vi "SetState.vi"(8 "Error In":errorcluster, 10 "State":bool, 11 "reference in":refnum<class "VdDigitalControl_DAQmx.lvclass">) -> (0 "Error Out":errorcluster, 3 "reference in":refnum<class "VdDigitalControl_DAQmx.lvclass">)   [LabVIEW 2020, in "VdDigitalControl_DAQmx.lvclass"]
uses:
  VdDigitalControl_DAQmx.lvclass
  <vilib>/DAQmx/write.llb/DAQmx Write (Digital Bool 1Line 1Point).vi
  <vilib>/DAQmx/miscellaneous.llb/DAQmx Fill In Error Info.vi
  VdDigitalControl_class/VdDigitalControl.lvclass
  VdDigitalControl_DAQmx.lvclass/VdDigitalControl_DAQmx.ctl
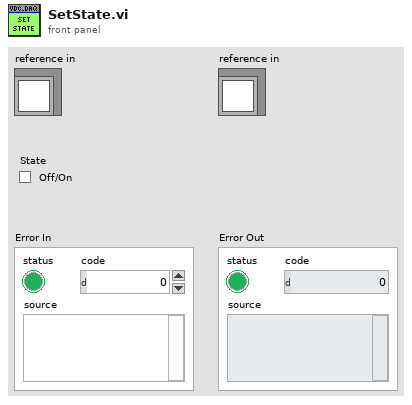
[diagram p1: front panel]
types:
  T1 = typedef "VdDigitalControl_DAQmx.lvclass/ObjectAttributes.ctl" = cluster{"task":refnum<k21>}
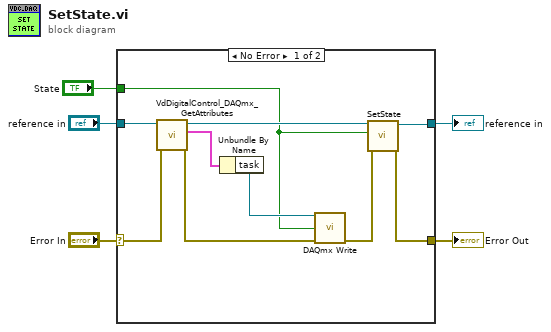
[diagram p0: block diagram]
diagram:
  n1 = case shown="No Error" "Error In" {
    selector: "Error In" -> [w7 w17]
    tunnel: [w11 w17] -> w4
    tunnel: [w12 w16] -> w2
    tunnel: "reference in" -> [w14 w16]
    tunnel: "State" -> [w8 _]
    frame No Error {
      n2 = call "VdDigitalControl_DAQmx_GetAttributes.vi"("error in (no error)"=w7, "reference in"=w14) -> ("error out"=w6:errorcluster, "Data"=w15:T1, "reference out"=w13:refnum<class "VdDigitalControl_DAQmx.lvclass">)  [unwired: 6 in, 1 out]
      n3 = Unbundle By Name(w15) -> ("task"=w10:refnum<k21>)
      n4 = call-poly <vilib>:"DAQmx Write.vi"("task/channels in"=w10, "data"=w8, "error in"=w6) -> ("error out"=w9:errorcluster)  [unwired: 10 in, 2 out]
      n5 = call-parent "SetState.vi"("Error In"=w9, "State"=w8, "reference in"=w13) -> ("Error Out"=w11:errorcluster, "reference in"=w12:refnum<class "VdDigitalControl_DAQmx.lvclass">)  [unwired: 7 in]
    }
    frame Error {
    }
  }
  "Error Out" <- w4
  "reference in" <- w2
